vi "ReversePal.vi"() -> ()   [LabVIEW 2015]
uses:
  <vilib>/sound2/lvsound2.llb/Sampling Mode.ctl
  <vilib>/sound2/lvsound2.llb/Sound Data Format.ctl
  <vilib>/sound2/lvsound2.llb/Sound Input Read (DBL).vi
panel:
  in  "stop":bool
  in  "number of samples/ch":i32=100000
  out "Señal Inversa":waveform(dbl)(graph)={"t0"=timestamp(0 s since 1904-01-01), "dt"=4.5e-05, "Y"=array[100000 elements]} caption="Signals"
  out "Señal Original":dynamicdata(graph)=[{"t0"=timestamp(0 s since 1904-01-01), "dt"=4.535147e-05, "Y"=array[100000 elements], "attributes"=variant("NI_ChannelName"=variant(string "Untitled"), "NI_ExpIsRelativeTime"=variant(bool TRUE), "NI_ExpStartTimeStamp"=variant(timestamp timestamp(3640469010.679152 s since 1904-01-01)), "NI_ExpTimeStamp"=variant(timestamp timestamp(3640469010.679152 s since 1904-01-01)), "NI_ExpXDimension"=variant(string "t"), "NI_UnitDescription"=variant(string "V"))}, {"t0"=timestamp(0 s since 1904-01-01), "dt"=4.535147e-05, "Y"=array[100000 elements], "attributes"=variant("NI_ChannelName"=variant(string "Untitled 1"), "NI_ExpIsRelativeTime"=variant(bool TRUE), "NI_ExpStartTimeStamp"=variant(timestamp timestamp(3640469010.679152 s since 1904-01-01)), "NI_ExpTimeStamp"=variant(timestamp timestamp(3640469010.679152 s since 1904-01-01)), "NI_ExpXDimension"=variant(string "t"), "NI_UnitDescription"=variant(string "V"))}] caption="Signals"
  # "Serrano Bermúdez Luis Esteban"
  # "Instrucciones de uso:"
  # "Para el funcionamiento de esta aplicación primero se debe grabar una pista primero, después detener la grabación\ny se pedirá un nombre para guardar los datos de la pista e inmediatamente la pista se reproducirá en orden  inverso a como fue grabada"
  # "11/05/2019"
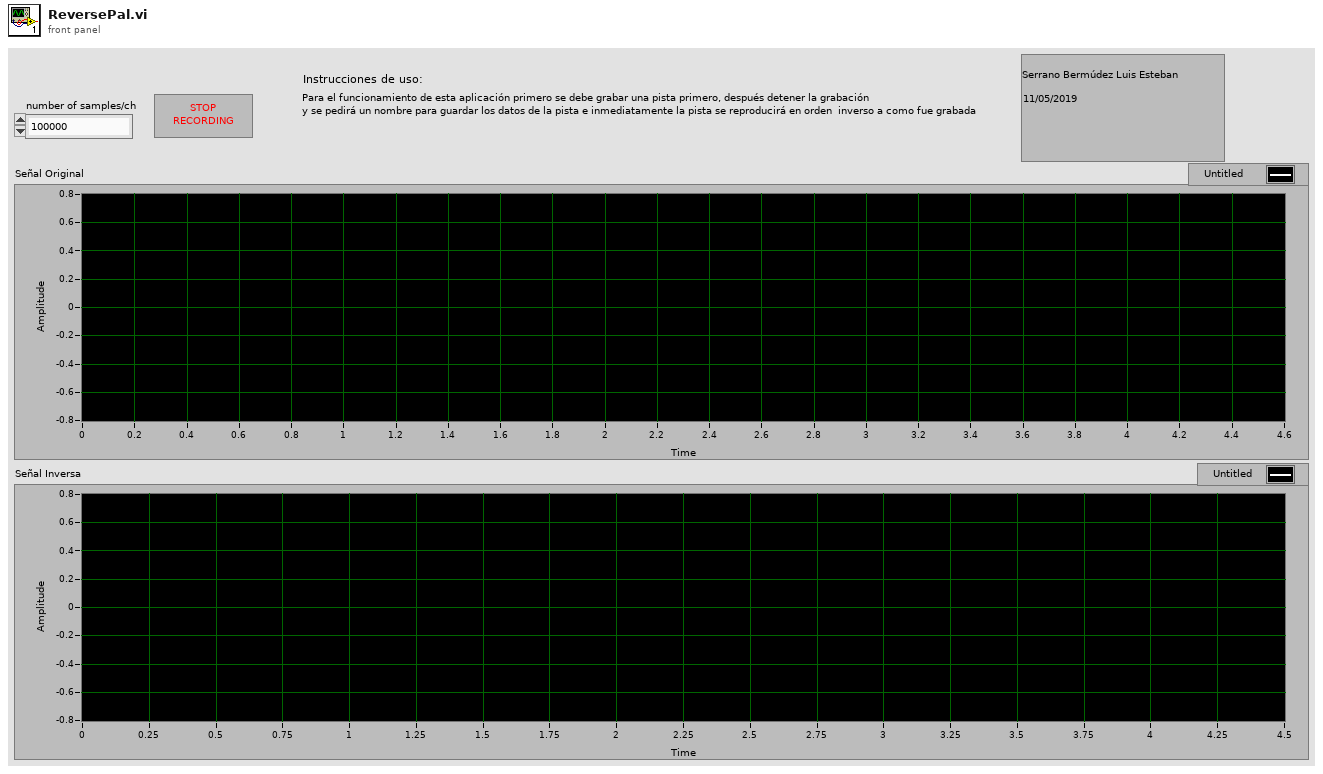
[diagram p1: front panel]
types:
  T1 = typedef "Sound Data Format.ctl" = cluster{"sample rate (S/s)":dbl, "number of channels":i32, "bits per sample":i32}
  T2 = typedef "Sampling Mode.ctl" = i32
  T3 = typedef "Sound Input Task ID.ctl" = u32
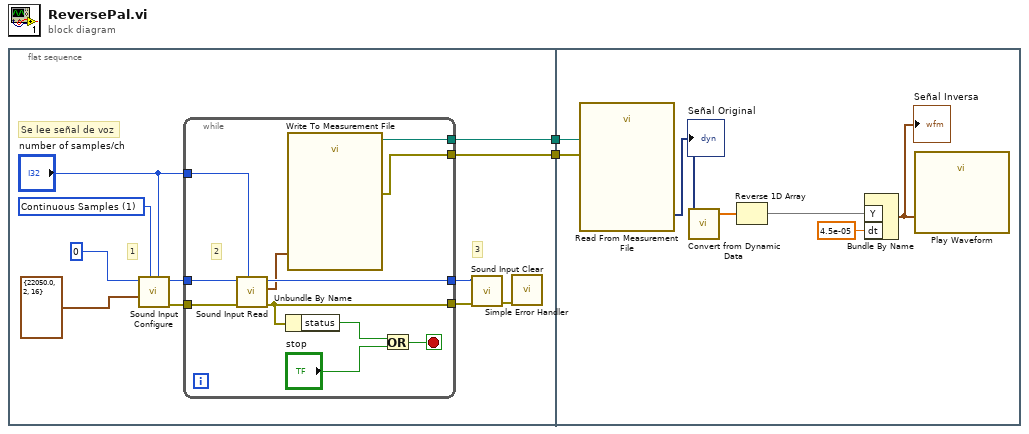
[diagram p0: block diagram]
diagram:
  n1 = flat-sequence {
    tunnel: [w5] -> w2
    tunnel: [w3] -> w1
    tunnel: w2 -> [w28]
    tunnel: w1 -> [w25]
    frame #0 {
      w6 = T2 1 items=["Finite Samples", "Continuous Samples"] ("sample mode")
      # "3"
      # "1"
      # "Se lee señal de voz"
      n2 = call <vilib>:"Sound Input Configure.vi"("number of samples/ch"="number of samples/ch", "sample mode"=w6, "sound format"=T1 {"sample rate (S/s)"=22050.0, "number of channels"=2, "bits per sample"=16}, "device ID"=u32 0) -> ("error out"=w9:errorcluster, "task ID"=w8:T3)  [unwired: 6 in]
      n3 = while {
        tunnel: w8 -> [w24]
        tunnel: w9 -> [w23]
        tunnel: "number of samples/ch" -> [w22]
        tunnel: [w21] -> w11
        tunnel: [w20] -> w12
        tunnel: [w15] -> w5
        tunnel: [w14] -> w3
        stop <- w17 stop-if-true
        # "2"
        n4 = call-poly <vilib>:"Sound Input Read.vi"("number of samples/ch"=w22, "error in (no error)"=w23, "task ID"=w24) -> ("error out"=w20:errorcluster, "data"=w16:waveform(dbl)[], "task ID out"=w21:T3)  [unwired: 6 in]
        n5 = Unbundle By Name(w20) -> ("status"=w19:bool)
        n6 = call "Write To Measurement File"("Signals"=w16) -> ("Filename Out"=w15:path, "error out"=w14:errorcluster)  [unwired: 16 in, 1 out]
        n7 = Or(x=w19, y="stop") -> (x .or. y?=w17:bool)
      }
      n8 = call <vilib>:"Sound Input Clear.vi"("error in (no error)"=w12, "task ID"=w11) -> ("error out"=w13:errorcluster)  [unwired: 9 in]
      n9 = call <vilib>:"Simple Error Handler.vi"("error in (no error)"=w13) -> ()  [unwired: 4 in, 5 out]
    }
    frame #1 {
      n10 = call "Read From Measurement File"("error in (no error)"=w25, "Filename"=w28) -> ("Signals"=w27:dynamicdata)  [unwired: 4 in, 5 out]
      "Señal Original" <- w27
      n11 = call "Convert from Dynamic Data"("Dynamic Data Type"=w27) -> ("Array"=w29:dbl[])  [unwired: 3 in]
      n12 = Reverse 1D Array(array=w29) -> (reversed array=w30:dbl[])
      n13 = Bundle By Name("Y"=w30, "dt"=4.5e-05) -> (w31:waveform(dbl))  [unwired: 1 in]
      "Señal Inversa" <- w31
      n14 = call "Play Waveform"("Data"=w31) -> ()  [unwired: 18 in, 1 out]
    }
  }
